vi "coordsRect.vi"(10 "Rozmiar":dbl, 11 "coords":cluster{"Width":dbl, "Height":dbl}) -> (3 "Cluster":cluster{dbl, dbl, dbl, dbl})   [LabVIEW 2020]
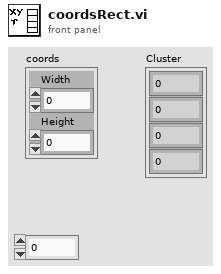
[diagram p1: front panel]
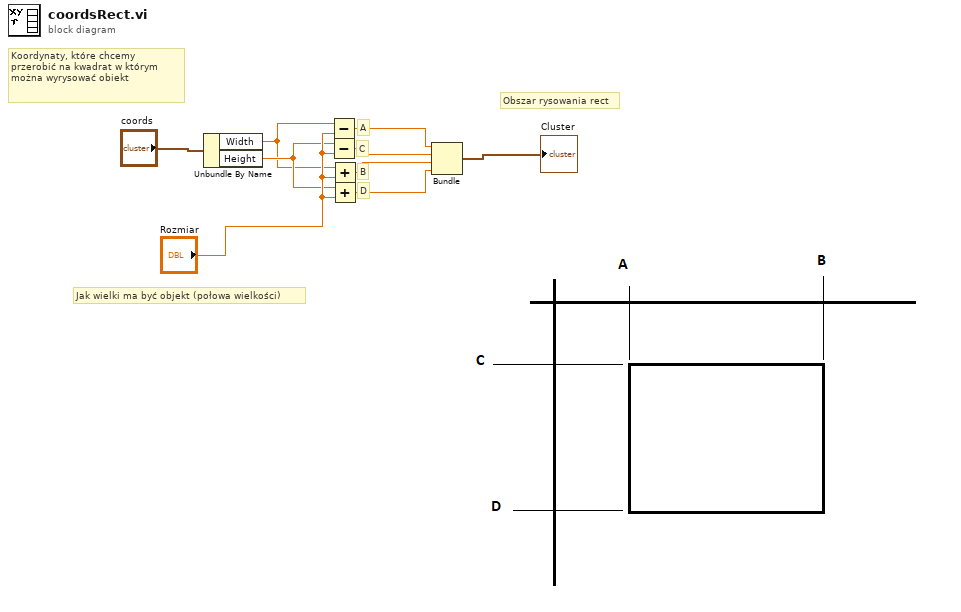
[diagram p0: block diagram]
diagram:
  # "D"
  # "C"
  # "B"
  # "A"
  # "Obszar rysowania rect"
  # "Jak wielki ma być objekt (połowa wielkości)"
  # "Koordynaty, które chcemy przerobić na kwadrat w którym można wyrysować obiekt"
  n1 = Unbundle By Name("coords") -> ("Width"=w5:dbl, "Height"=w6:dbl)
  n2 = Subtract(x=w5, y="Rozmiar") -> (x-y=w1:dbl)
  n3 = Subtract(x=w6, y="Rozmiar") -> (x-y=w2:dbl)
  n4 = Add(x=w5, y="Rozmiar") -> (x+y=w3:dbl)
  n5 = Add(x=w6, y="Rozmiar") -> (x+y=w4:dbl)
  n6 = Bundle(w1, w2, w3, w4) -> (→"Cluster":cluster{dbl, dbl, dbl, dbl})  [unwired: 1 in]
